vi "Configure IF Gain.vi"   [LabVIEW 2018, in "Agilent MXA Series.lvlib"]
doc: "Configures the IF gain."
uses:
  Agilent MXA Series.lvlib
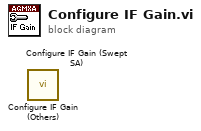
[diagram p0: block diagram]
diagram:
  n1 = call "Configure IF Gain (Others).vi"() -> ()  [unwired: 10 in, 2 out]
  n2 = call "Configure IF Gain (Swept SA).vi"() -> ()  [unwired: 10 in, 2 out]
